vi "Thumbnails.vi"(6 "Digitizer Settings":T1={"Digitizer delay (us) "=0.0, "rf points per line"=2048, "lines per plane"=128, "Samp Rate (Hz)"=100000000.0, "Additional dig delay (us)"=0.0, "Voltage Scale"=0.4, "Pre-Looks"=0, "Offset delay (us)"=0.0, "bits A/D"=8, "Avg Num"=1, "DigTimeOut"=5.0, "Rel Dig Delay"=0.0, "Dig Ch"=0, "LeCroyCluster"={"LeCroy Channels"=[TRUE, FALSE, FALSE, FALSE], "LC read pt offset"=0.0, "Sweep Avg"=FALSE}, "Main Digitizer"=enum."NI Digitizer", "Dig Config"=enum."Single channel", "Digitizer ID Cluster"={"Acqiris/Alazar/SP ID"=[], "NI Instr Handles"=[], "LeCroy VISA"="", "GaGe Handle"={"Handle"=0, "Sample size"=0, "Resolution"=0, "Offset"=0, "Channels"=0, "Boards"=0}, "ATS Ref"="ATS9350", "Acqiris Address"=["PCI::INSTR0"], "ADQRef"=refnum, "adq_cu_ptr"=refnum}, "Trigger Settings"={"Trig Source"=1, "Trig Coupling"=0, "Trig Slope"=0, "Level (mV)"=1500.0}, "Bulk Acq"=FALSE, "Bulk Start Indexes"=[], "Data Ref RF"=refnum, "NI ID/Channel"=[], "Total Dig CH"=1, "Xtra Ann Trig delay (us)"=10.0, "Fix Z Delay?"=FALSE, "One Way Transmission?"=FALSE, "Data Ref Log"=refnum} {"Trigger Settings"."Trig Slope" items=["Positive", "Negative"]; "Trigger Settings"."Level (mV)" format="%.2f"; "Trigger Settings"."Trig Coupling" items=["DC 1 MOhm", "AC 1 MOhm", "DC 50 Ohm", "AC 50 Ohm"]; "Trigger Settings"."Trig Source" items=["Chan 1", "External"]; "Rel Dig Delay" format="%.2f"; "DigTimeOut" format="%.2f"; "Avg Num" min=1; "Offset delay (us)" format="%.2f"; "Additional dig delay (us)" format="%.2f"; "Digitizer delay (us)" format="%.2f"}, 8 "pixels in y":i16=180, 9 "pixels in x":i16=200) -> (2 "Thumb Size":cluster{"pixels in x":i16, "pixels in y":i16}, 3 "Thumbs out":picture[](array[picture]))   [LabVIEW 2022 SP3]
uses:
  Digitizers/-DigitizerRoutines/DigitizerSettings.ctl
  Digitizers/-DigitizerRoutines/Digitizer.ctl
  Digitizers/-DigitizerRoutines/DigConfig.ctl
  Digitizers/-DigitizerRoutines/DigitizerID.ctl
  C:/Windows/System32/ADQAPI_dotNet_helper.dll
  Motion Controllers/-MotionRoutines/MotionGlobals.vi
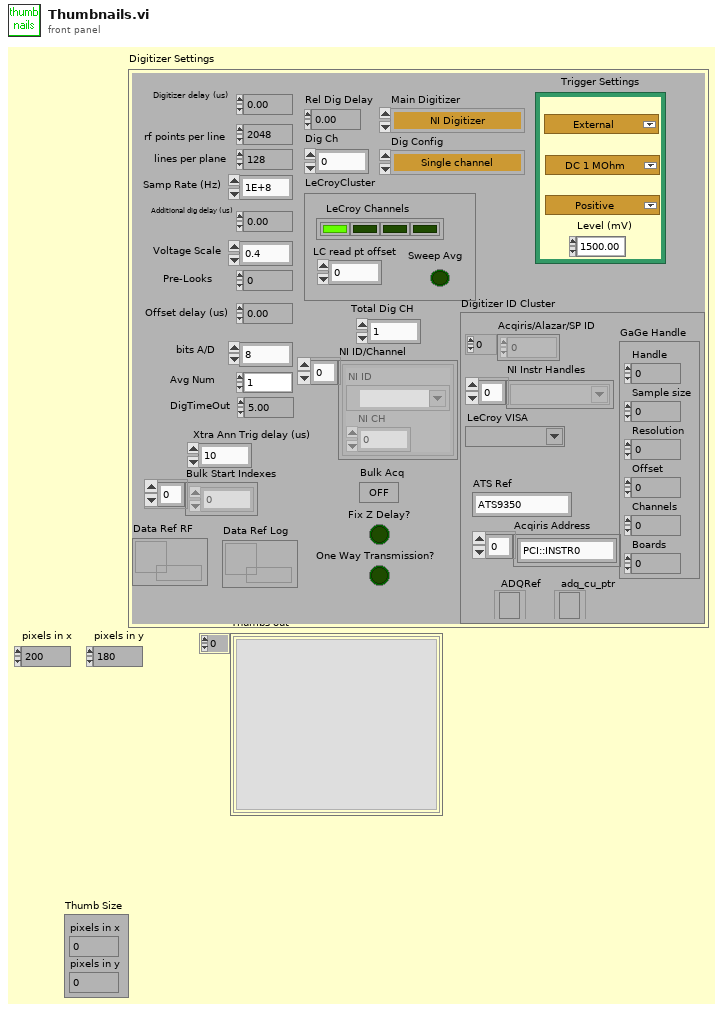
[diagram p1: front panel]
types:
  T1 = typedef "DigitizerSettings.ctl" = cluster{"Digitizer delay (us) ":dbl, "rf points per line":i32, "lines per plane":i32, "Samp Rate (Hz)":dbl, "Additional dig delay (us)":dbl, "Voltage Scale":dbl, "Pre-Looks":i32, "Offset delay (us)":dbl, "bits A/D":i8, "Avg Num":i32, "DigTimeOut":sgl, "Rel Dig Delay":sgl, "Dig Ch":i32, "LeCroyCluster":cluster{"LeCroy Channels":bool[], "LC read pt offset":dbl, "Sweep Avg":bool}, "Main Digitizer":T2, "Dig Config":T3, "Digitizer ID Cluster":T4, "Trigger Settings":cluster{"Trig Source":u16, "Trig Coupling":u16, "Trig Slope":u16, "Level (mV)":dbl}, "Bulk Acq":bool, "Bulk Start Indexes":i32[], "Data Ref RF":refnum<data-value>, "NI ID/Channel":cluster{"NI ID":refnum<k15>, "NI CH":i32}[], "Total Dig CH":i32, "Xtra Ann Trig delay (us)":dbl, "Fix Z Delay?":bool, "One Way Transmission?":bool, "Data Ref Log":refnum<data-value>}
  T2 = typedef "Digitizer.ctl" = enum16{"Acqiris Digitizer", "NI Digitizer", "LeCroy", "GaGe", "AlazarTech", "No Digitizer", "Teledyne"}
  T3 = typedef "DigConfig.ctl" = enum16{"Single channel", "2 Chans w/ 2 Acqiris", "2 Chans w/ 1 Acqiris", "5-CH Pulser New", "5-CH pulser w/ ann array", "5-pass style ann array", "Empty"}
  T4 = typedef "DigitizerID.ctl" = cluster{"Acqiris/Alazar/SP ID":u32[], "NI Instr Handles":refnum<k15>[], "LeCroy VISA":refnum<visa-resource-name>, "GaGe Handle":cluster{"Handle":u32, "Sample size":u32, "Resolution":i32, "Offset":i32, "Channels":u32, "Boards":u32}, "ATS Ref":string, "Acqiris Address":string[], "ADQRef":refnum<k24>, "adq_cu_ptr":refnum<k24>}
  T5 = cluster{"Font Name:":string, "Size":i16, "Strikeout?":bool, "Italic?":bool, "Underline?":bool, "Outline?":bool, "Shadow?":bool, "Bold?":bool}
  T6 = typedef "Header.ctl" = cluster{"header info":cluster{"Header":string, "Head length":i16}, "A/D info":cluster{"# rf points per line":u16, "# lines per scan":u16, "sample rate MHz":u16, "# A/D bits":i16, "# bytes per A/D":u16, "TGC Flag":u16, "A/D Type":string}, "Tranducer Info":cluster{"bandwidth":sgl, "center freq":sgl, "start freq":sgl, "ID":i32}, "Scan Info":cluster{"delay":sgl, "pivot distance":sgl, "sector scan angle":sgl, "operator":string, "Scan Mode":string, "location":string}, "Time/Date Info":cluster{"date":string, "time":string}, "RF Info":cluster{"RF file name":string, "RF file att":string, "RF cal file name":string, "RF cal file att":string}, "Patient Info":cluster{"ID":string, "extended ID":string, "age":u16, "sex":string, "previously\nscanned":string, "PSA":sgl, "LOS":u8, "Ethnicty 2":u8, "Race":u8}, "Tissue Type":cluster{"organ":i16, "disease type":i16, "disease location":i16, "IQ_pts":u16, "RcvBuffer":u8, "RcvFrame":u16, "IQBuff":u8, "IQFrame":u16, "IQPage":u8}, "Votage scaling":cluster{"Digitizer (dB)":sgl, "Gain (dB)":sgl, "Atten (dB)":sgl}, "Comment":string, "Misc Info":cluster{"avg num":u16, "c speed":i16, "Div By or SF zones":i16, "XMIT CHS":u8, "RCV CHS":u8, "Xmit angle":sgl}, "Therapy Parameters":cluster{"Theraputic Freq (MHz)":sgl, "Time on (s)":sgl, "Therapy amplitude (mV)":sgl, "Lines Before":u16, "Lines After":u16}, "Scan Settings":cluster{"Energy (uJ or V)":u8, "Damp (Ohm) or Fc":u8, "HP Filt (KHz)":u8, "LP Filt (MHz)":u8, "Gain (db)":u8, "prf (kHz)":sgl, "Distance between\nscan lines (um)":u16, "Distance between\nscan planes (um)":u16, "Scan line gap (um)":sgl, "Scan plane gap (um)":sgl}, "Compression Parameters":cluster{"F1 (MHz)":sgl, "F2 (MHz)":sgl, "% taper":sgl, "duration":sgl}, "Patient Info Xtra":cluster{"First Name":string, "Last Name":string, "Notes":string}, "ROI Box":u16[]}
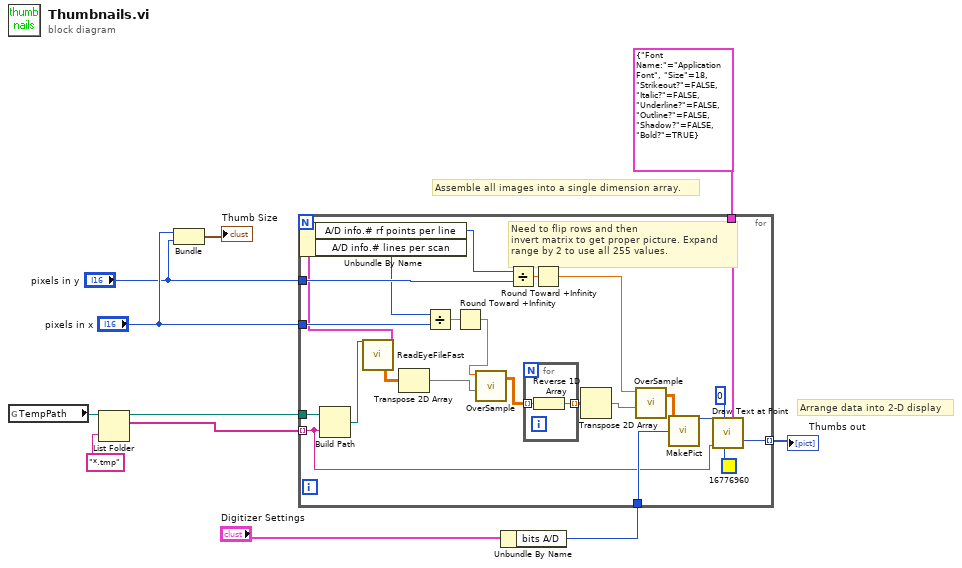
[diagram p0: block diagram]
diagram:
  # "Arrange data into 2-D display"
  # "Assemble all images into a single dimension array."
  n1 = global read "MotionGlobals.vi" "TempPath"() -> (w3:path)
  n2 = List Folder(path=w3, pattern="*.tmp") -> (path out=w6:path, filenames=w7:string[])  [unwired: 1 in, 3 out]
  n3 = Bundle("pixels in x"="pixels in x", "pixels in y"="pixels in y") -> (→"Thumb Size":cluster{"pixels in x":i16, "pixels in y":i16})  [unwired: 1 out]
  n4 = Unbundle By Name("Digitizer Settings") -> ("bits A/D"=w2:i8)
  n5 = for {
    tunnel: [w32] -> w11 mode=indexing
    tunnel: T5 {"Font Name:"="Application Font", "Size"=18, "Strikeout?"=FALSE, "Italic?"=FALSE, "Underline?"=FALSE, "Outline?"=FALSE, "Shadow?"=FALSE, "Bold?"=TRUE} ("[user-specified font]") -> [w31]
    tunnel: w2 -> [w29]
    tunnel: w7 -> [w24] mode=indexing
    tunnel: w6 -> [w28]
    tunnel: "pixels in x" -> [w23]
    tunnel: "pixels in y" -> [w21]
    # "Need to flip rows and then\ninvert matrix to get proper picture. Expand \nrange by 2 to use all 255 values."
    n6 = Build Path(base path=w28, name or relative path=w24) -> (appended path=w27:path)
    n7 = call "ReadEyeFileFast.vi"("new file path"=w27) -> ("2-D data array"=w26:sgl[][], "Header In"=w14:T6)  [unwired: 1 in, 16 out]
    n8 = Unbundle By Name(w14) -> ("A/D info.# rf points per line"=w13:u16, "A/D info.# lines per scan"=w12:u16)
    n9 = Transpose 2D Array(2D array=w26) -> (transposed array=w19:sgl[][])
    n10 = Divide(x=w12, y=w23) -> (x/y=w25:dbl)
    n11 = Round Toward +Infinity(x=w25) -> (ceil(x): smallest int >= x=w20:dbl)
    n12 = call "OverSample.vi"("raw data in"=w19, "reduce RF pts by factor of"=w20) -> ("reduced data out"=w18:dbl[][])  [unwired: 3 in]
    n13 = Divide(x=w13, y=w21) -> (x/y=w22:dbl)
    n14 = for {
      tunnel: w18 -> [w37] mode=indexing
      tunnel: [w36] -> w33 mode=indexing
      n15 = Reverse 1D Array(array=w37) -> (reversed array=w36:dbl[])
    }
    n16 = Round Toward +Infinity(x=w22) -> (ceil(x): smallest int >= x=w16:dbl)
    n17 = Transpose 2D Array(2D array=w33) -> (transposed array=w17:dbl[][])
    n18 = call "OverSample.vi"("raw data in"=w17, "reduce RF pts by factor of"=w16) -> ("reduced data out"=w15:dbl[][])  [unwired: 3 in]
    n19 = call "MakePict.vi"("lower dB limit"=w29, "raw data in"=w15) -> ("new picture"=w35:picture)  [unwired: 1 in, 2 out]
    n20 = call <vilib>:"Draw Text at Point.vi"("[user-specified font]"=w31, "text color(black)"=u32 16776960, "desired font(Application)"=0, "text"=w24, "picture"=w35) -> ("new picture"=w32:picture)  [unwired: 4 in, 2 out]
  }
  "Thumbs out" <- w11
